vi "ADC Converter.vi"(8 "error in":errorcluster, 11 "ADC in":u32) -> (0 "error out":errorcluster, 3 "ADC out":dbl)   [LabVIEW 2019, in "LED.lvlib"]
uses:
  LED/LED.lvlib
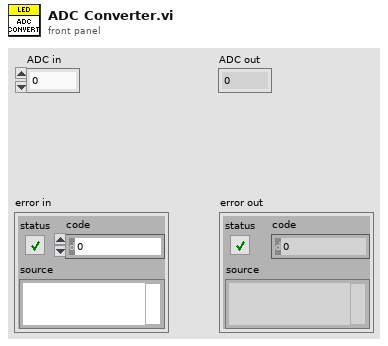
[diagram p1: front panel]
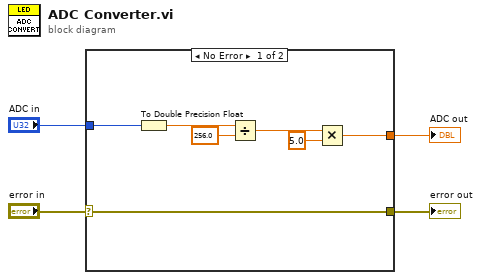
[diagram p0: block diagram]
diagram:
  n1 = case shown="No Error" "error in" {
    selector: "error in" -> [w5 w12]
    tunnel: "ADC in" -> [w11 _]
    tunnel: [w6 _] -> w3
    tunnel: [w5 w12] -> w1
    frame No Error {
      n2 = To Double Precision Float(number=w11) -> (double precision float=w10:dbl)
      n3 = Divide(x=w10, y=256.0) -> (x/y=w8:dbl)
      n4 = Multiply(x=w8, y=5.0) -> (x*y=w6:dbl)
    }
    frame Error {
    }
  }
  "ADC out" <- w3
  "error out" <- w1
